vi "Read State from File.vi"(0 "Display State In":T1, 5 "tdms file":refnum<k34>, 7 "Lable.Text":string, 9 "Container State":T2, 11 "error in (no error)":errorcluster) -> (4 "Display State Out":T1, 6 "tdms file out":refnum<k34>, 15 "error out":errorcluster)   [LabVIEW 2015, in "Dynamic FP XControl.xctl"]
uses:
  Dynamic FP XControl.xctl
  <vilib>/_xctls/Container State.ctl
  Dynamic FP container.llb/Dynamic FP State.ctl
  Device/Device.lvclass
  Name type and data.ctl
  Device/Device type.ctl
  <vilib>/_xctls/XControlSupport.lvlib
panel:
  # "Add Controls & Indicators that form the parameters of the method here. Hook them to the connector pane. Do not delete the controls & indicators that are already hooked to the connector pane.\n \nTo setup the parameters  for this method, right click on this item in the Project Tree & select \"Configure Method...\"."
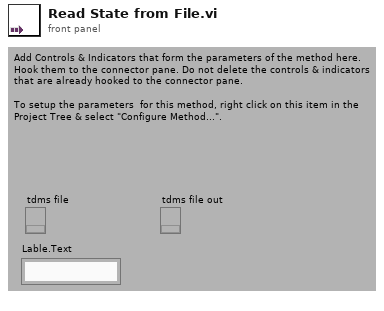
[diagram p1: front panel]
types:
  T1 = typedef "Dynamic FP XControl.xctl/Dynamic FP State.ctl" = cluster{"Complete device list":refnum<class "Device.lvclass">[], "Boolean test":bool, "Selected devices":u16[]}
  T2 = typedef "XControlSupport.lvlib/Container State.ctl" = cluster{"Indicator?":bool, "Run Mode?":bool, " Refnum":refnum<vi>}
  T3 = typedef "Name type and data.ctl" = cluster{"Front Panel Data":variant, "Device type":T4, "Name":string}
  T4 = typedef "Device type.ctl" = enum16{"NONE", "Neocera 21", "LakeShore 335", "LakeShore 340", "LkShr 340 chA&B", "LakeShore 370", "SRS 850", "SRS 830", "LR 700", "EG&G 5302", "EG&G 7260", "EG&G 7280", "AH 2500", "Keithley meter", "Keithley electrometer", "Keithley 182", "HP 5385", "HP 53181", "HP 53132", "ITC503", "IPS120", "Oxford Mercury IPS", "Oxford PS", "Test", "DC Facility Magnet", "Cryomagnetics PS", "Keithley 2400", "Keithley current source", "Cryo-Con 22C", "HP87NN", "HP4395A"}
  T5 = cluster{"Saved device":i32, "Present device":i32}[]
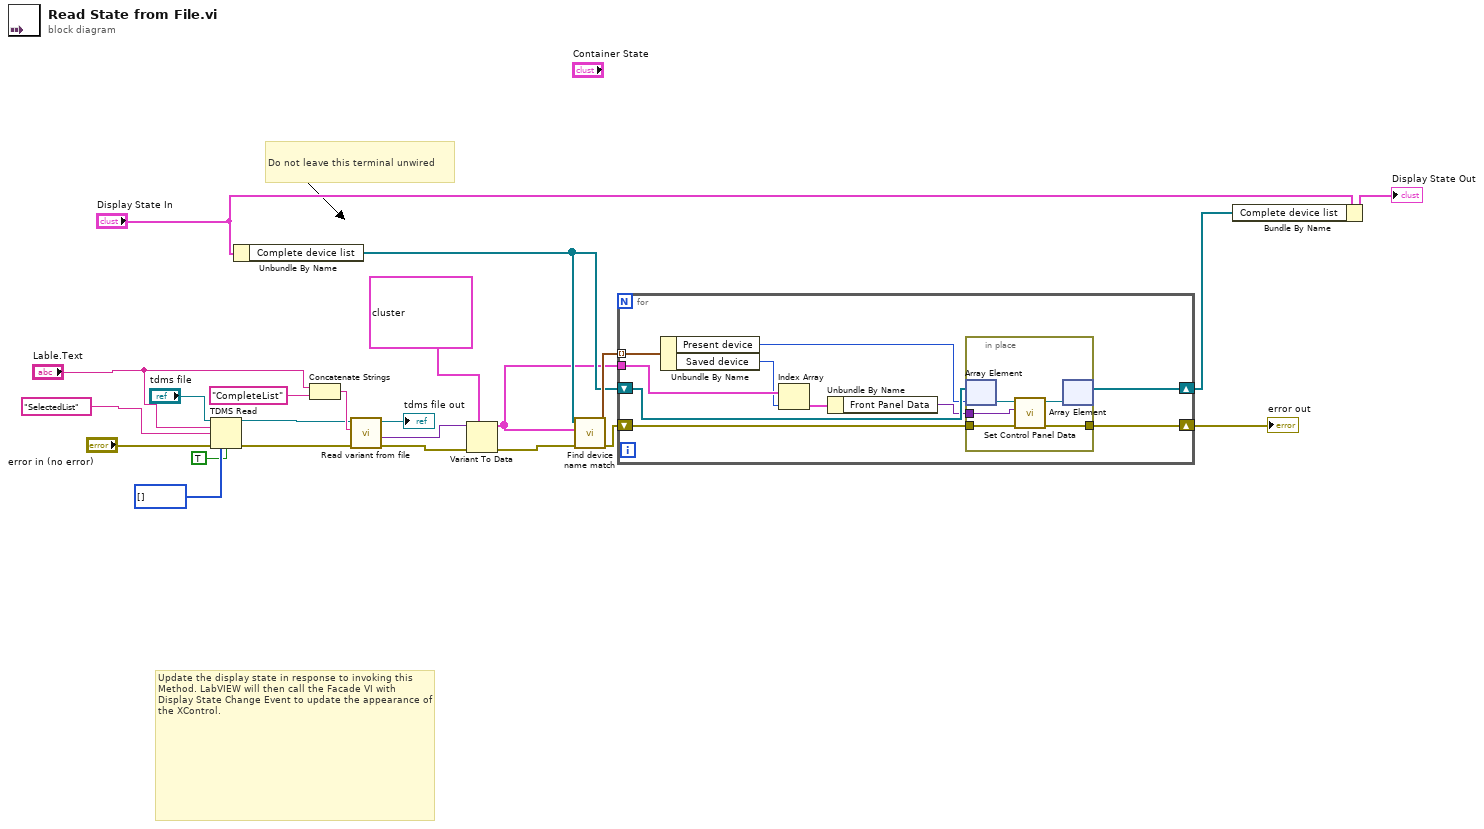
[diagram p0: block diagram]
diagram:
  # "Do not leave this terminal unwired"
  # "Update the display state in response to invoking this Method. LabVIEW will then call the Facade VI with Display State Change Event to update the appearance of the XControl."
  n1 = TDMS Read(0:"tdms file", 5:"Lable.Text", 7:"SelectedList" ("string"), 11:"error in (no error)", 12:u16[] [] ("Selected devices"), 13:TRUE ("return channels in file order? (F)")) -> (4:w18:refnum<k34>, 15:w19:errorcluster)  [unwired: 2 in, 4 out]
  n2 = Unbundle By Name("Display State In") -> ("Complete device list"=w7:refnum<class "Device.lvclass">[])
  n3 = Concatenate Strings("Lable.Text", "CompleteList" ("string")) -> (w20:string)
  n4 = call "Read variant from file.vi"("error in (no error)"=w19, "group name in"=w20, "tdms file"=w18) -> ("error out"=w13:errorcluster, "variant out"=w15:variant, "tdms file out"=→"tdms file out":refnum<k34>)  [unwired: 6 in]
  n5 = Variant To Data(error in=w13, type=T3[] [{"Front Panel Data"=variant, "Device type"=enum."NONE", "Name"=""}], Variant=w15) -> (data=w6:T3[], error out=w9:errorcluster)
  n6 = call "Find device name match.vi"("error in"=w9, "Saved names and data"=w6, "Device list"=w7) -> ("error out"=w5:errorcluster, "Matching pairs"=w8:T5)  [unwired: 7 in]
  n7 = for {
    tunnel: w8 -> [w32] mode=indexing
    shift-right: [w28] -> w3
    shift-left: w7 -> [w33]
    tunnel: w6 -> [w30]
    shift-right: [w25] -> w2
    shift-left: w5 -> [w26]
    n8 = Unbundle By Name(w32) -> ("Present device"=w31:i32, "Saved device"=w29:i32)
    n9 = Index Array(array=w30, index=w29) -> (element=w27:T3)
    n10 = Unbundle By Name(w27) -> ("Front Panel Data"=w24:variant)
    n11 = in-place {
      in-place-border: w24 -> [w36]
      in-place-border: w26 -> [w35]
      in-place-border: [w34] -> w25
      n12 = in-place-array #1(w33, w31) -> (w38:refnum<class "Device.lvclass">)
      n13 = call "Set Control Panel Data.vi"("error in (no error)"=w35, "Data"=w36, "Device in"=w38) -> ("error out"=w34:errorcluster, "Device out"=w37:refnum<class "Device.lvclass">)  [unwired: 7 in]
      n14 = in-place-array #1(w37) -> (w28:refnum<class "Device.lvclass">[])  [unwired: 1 out]
    }
  }
  "error out" <- w2
  n15 = Bundle By Name(cluster="Display State In", "Complete device list"=w3) -> (→"Display State Out":T1)
